vi "Calculate Assign Pt Demo.vi"(8 "Deform Array":dbl[](array[numeric])=[1.0, 1.0, 1.0, 0.0, 0.0, 0.0, 0.0, 0.0, 0.0], 9 "Eye Model Cluster":T2={"X Grid"=[], "Y Grid"=[], "Za_true Surf"=[], "Iris Center"=[], "Zp_true Surf"=[], "Pinv"=[[1.0, 0.0], [0.0, 1.0]], "za_true"=5.0, "za_work"=1.0, "zp_work"=-1.0, "zp_true"=-5.0}, 10 "Assign Pt":dbl[](array[numeric])=[0.0, 5.0, 0.0], 11 "Current Pt":dbl[](array[numeric])=[0.0, 0.0, 0.0]) -> (0 "Assign Pt OOB":bool, 3 "Assign Pt*":dbl[](array[numeric]))   [LabVIEW 2016]
uses:
  <vilib>/Analysis/Matrix/Datatypes/RealMatrix.ctl
  <vilib>/Analysis/_algsub.llb/Vector Norm Type.ctl
  <vilib>/Analysis/baseanly.llb/A x Vector.vi
  <vilib>/Analysis/_algsub.llb/Real Vector Norm.vi
  Subsystems/Global Variables.vi
  <vilib>/Analysis/7linalg.llb/Create Special Real Matrix.vi
  <vilib>/Analysis/baseanly.llb/Real Inverse Matrix.vi
  <vilib>/Analysis/NI_AALBase.lvlib
  <vilib>/Analysis/NI_AALPro.lvlib
  <vilib>/Analysis/NI_AALBLAS.lvlib
  <vilib>/Analysis/Matrix/NI_Matrix.lvlib
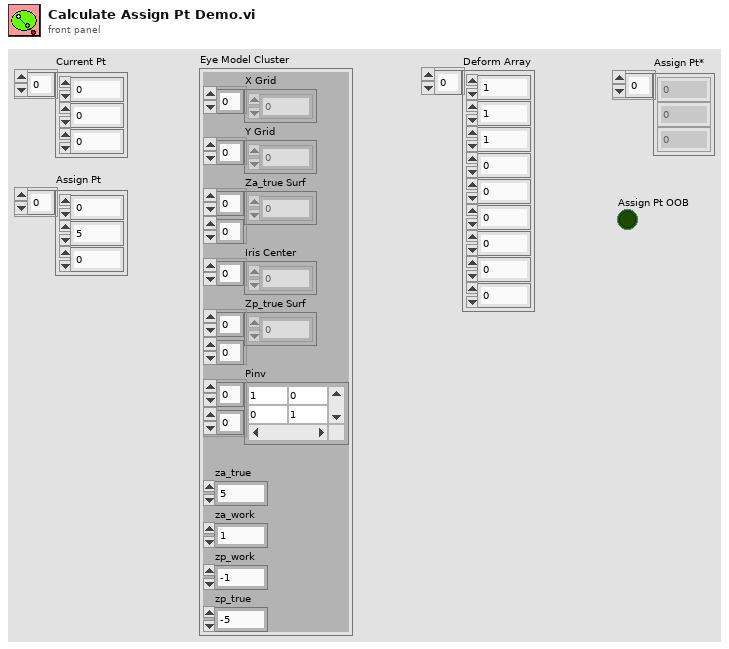
[diagram p1: front panel]
types:
  T1 = typedef "NI_Matrix.lvlib/RealMatrix.ctl" = dbl[][]
  T2 = cluster{"X Grid":dbl[], "Y Grid":dbl[], "Za_true Surf":dbl[][], "Iris Center":dbl[], "Zp_true Surf":dbl[][], "Pinv":T1, "za_true":dbl, "za_work":dbl, "zp_work":dbl, "zp_true":dbl}
  T3 = typedef "NI_AALPro.lvlib/Vector Norm Type.ctl" = u16
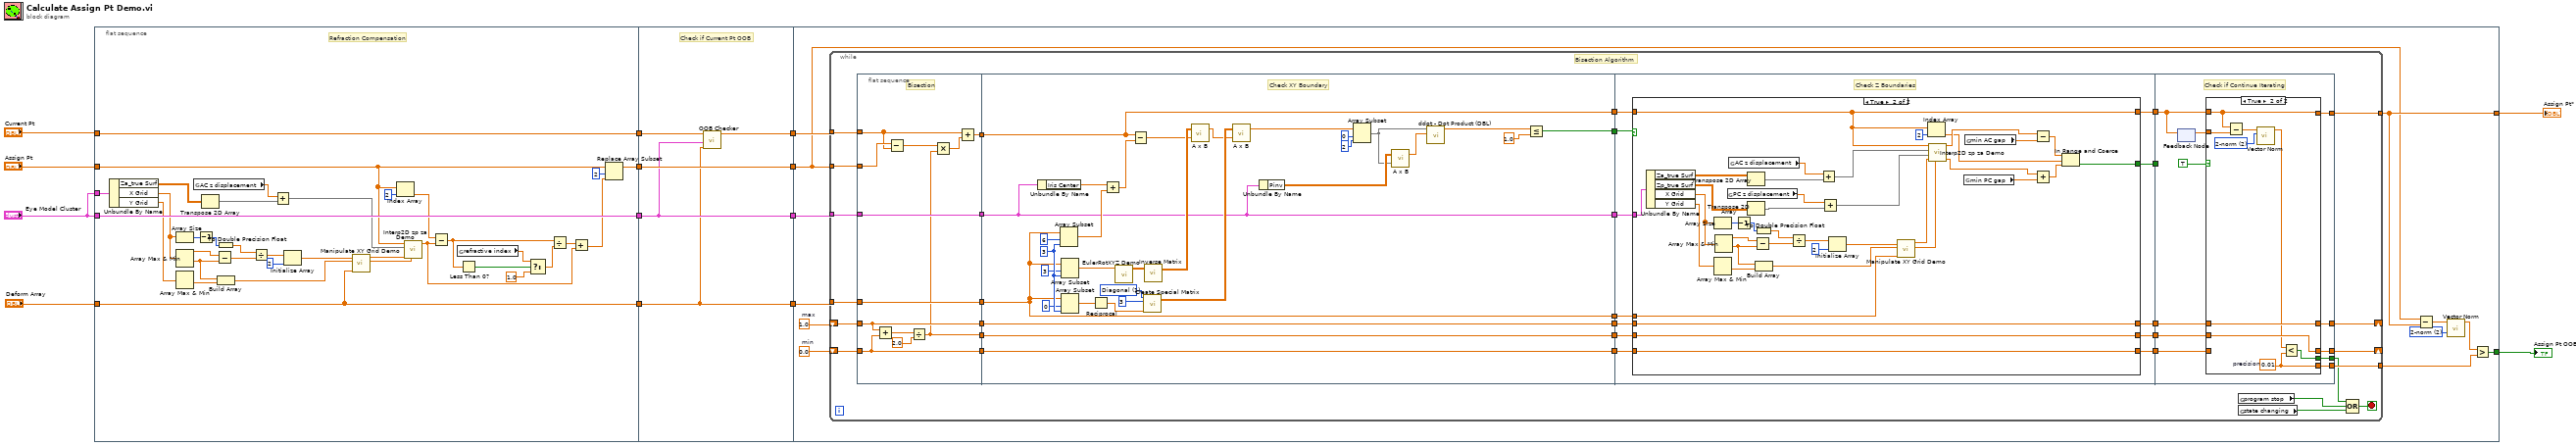
[diagram p0: block diagram]
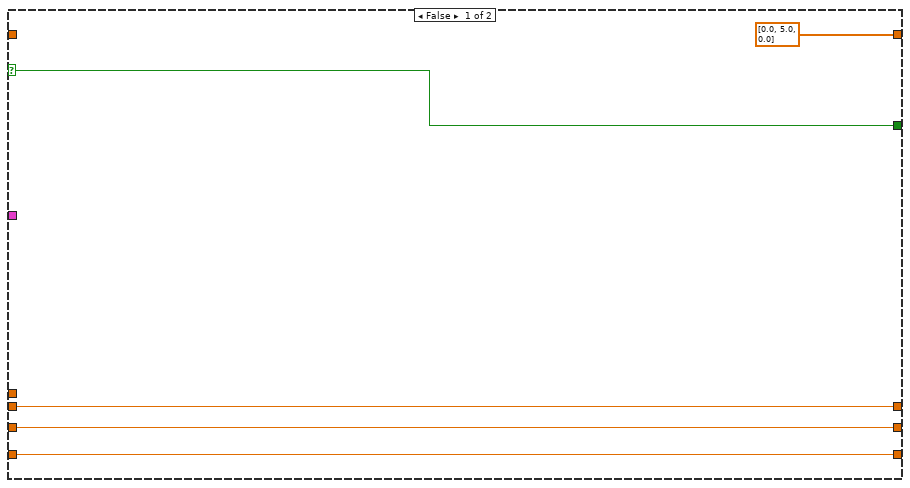
[diagram p2: hidden frame]
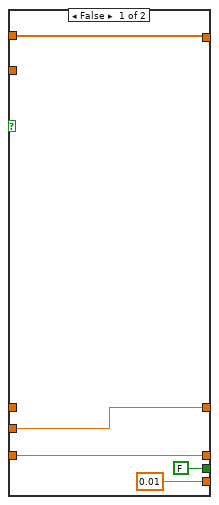
[diagram p3: hidden frame]
diagram:
  n1 = flat-sequence {
    tunnel: "Current Pt" -> [w28]
    tunnel: "Deform Array" -> [w30]
    tunnel: "Eye Model Cluster" -> [w50]
    tunnel: "Assign Pt" -> [w22]
    tunnel: [w23] -> w9
    tunnel: [w50] -> w7
    tunnel: [w30] -> w5
    tunnel: [w28] -> w3
    tunnel: "Eye Model Cluster" -> [w31]
    tunnel: w9 -> [w55]
    tunnel: [w55] -> w8
    tunnel: w7 -> [w52]
    tunnel: [w52] -> w6
    tunnel: w5 -> [w51]
    tunnel: [w51] -> w4
    tunnel: w3 -> [w54]
    tunnel: [w53] -> w2
    tunnel: w8 -> [w57]
    tunnel: w6 -> [w66]
    tunnel: w4 -> [w65]
    tunnel: w2 -> [w64]
    tunnel: [w60] -> w10
    tunnel: [w61] -> w1
    frame #0 {
      # "Refraction Compensation"
      n2 = Unbundle By Name(w31) -> ("Za_true Surf"=w34:dbl[][], "X Grid"=w46:dbl[], "Y Grid"=w47:dbl[])
      n3 = Array Size(array=w46) -> (size(s)=w39:i32)
      n4 = Array Max & Min(array=w46) -> (max value=w41:dbl, min value=w40:dbl)  [unwired: 2 out]
      n5 = Array Max & Min(array=w47) -> (min value=w42:dbl)  [unwired: 3 out]
      n6 = global read "Global Variables.vi" "AC z displacement"() -> (w33:dbl)
      n7 = Decrement(x=w39) -> (x-1=w44:i32)
      n8 = Transpose 2D Array(2D array=w34) -> (transposed array=w32:dbl[][])
      n9 = Subtract(x=w41, y=w40) -> (x-y=w45:dbl)
      n10 = To Double Precision Float(number=w44) -> (double precision float=w43:dbl)
      n11 = Build Array(w40, w42) -> (w35:dbl[])
      n12 = Divide(x=w43, y=w45) -> (x/y=w37:dbl)
      n13 = Add(x=w33, y=w32) -> (x+y=w29:dbl[][])
      n14 = Initialize Array(w37, 2 ("dimension size")) -> (w36:dbl[])
      n15 = call "Manipulate XY Grid Demo.vi"("Deform Array"=w30, "XY Grid min In"=w35, "XY Quant. Fact. In"=w36) -> ("XY Grid min Out"=w49:dbl[], "XY Quant. Fact. Out"=w48:dbl[])  [unwired: 7 in]
      n16 = Index Array(array=w22, index=2) -> (element=w26:dbl)
      n17 = call "Interp2D zp za Demo.vi"("XY Grid min"=w49, "XY Quantization Factor"=w48, "Za array"=w29, "Tip Position"=w22) -> ("za"=w25:dbl)  [unwired: 6 in, 1 out]
      n18 = Subtract(x=w26, y=w25) -> (x-y=w16:dbl)
      n19 = global read "Global Variables.vi" "refractive index"() -> (w18:dbl)
      n20 = Less Than 0?(x=w16) -> (x < 0?=w19:bool)
      n21 = Select(t=w18, s=w19, f=1.0) -> (s? t:f=w15:dbl)
      n22 = Divide(x=w16, y=w15) -> (x/y=w24:dbl)
      n23 = Add(x=w24, y=w25) -> (x+y=w20:dbl)
      n24 = Replace Array Subset(array=w22, new element=w20, index=2) -> (w23:dbl[])
    }
    frame #1 {
      # "Check if Current Pt OOB"
      n25 = call "OOB Checker.vi"("Deform Array"=w51, "Eye Model Cluster"=w52, "Check Pt"=w54) -> ("Check Pt*"=w53:dbl[])  [unwired: 7 in, 1 out]
    }
    frame #2 {
      w58 = T3 2 items=["1-norm"=1, "2-norm"=2, "Inf-norm"=3, "-Inf-norm"=4, "User Defined"=5] ("norm type")
      w67 = 0.0  # min
      w63 = 1.0  # max
      n26 = while {
        tunnel: w64 -> [w97]
        shift-right: [w80] -> _
        shift-left: w63 -> [w99]
        shift-right: [w78] -> _
        shift-left: w67 -> [w98]
        tunnel: w57 -> [w96]
        tunnel: w66 -> [w91]
        tunnel: w65 -> [w90]
        tunnel: [w73] -> w60
        tunnel: [w72] -> w62
        stop <- w71 stop-if-true
        # "Bisection Algorithm"
        n27 = flat-sequence {
          tunnel: [w107] -> w95
          tunnel: [w104] -> w94
          tunnel: [w103] -> w93
          tunnel: [w102] -> w92
          tunnel: [w101] -> w89
          tunnel: w99 -> [w104]
          tunnel: w98 -> [w103]
          tunnel: w97 -> [w108]
          tunnel: w96 -> [w109]
          tunnel: w91 -> [w102]
          tunnel: w90 -> [w101]
          tunnel: [w100] -> w77
          tunnel: w95 -> [w115]
          tunnel: w94 -> [w122]
          tunnel: w93 -> [w121]
          tunnel: w92 -> [w114]
          tunnel: w89 -> [w113]
          tunnel: [w123] -> w88
          tunnel: [w122] -> w87
          tunnel: [w121] -> w86
          tunnel: [w115] -> w85
          tunnel: [w114] -> w84
          tunnel: [w113] -> w83
          tunnel: w77 -> [w112]
          tunnel: [w112] -> w76
          tunnel: w88 -> [w155]
          tunnel: w87 -> [w154]
          tunnel: w86 -> [w153]
          tunnel: w85 -> [w151]
          tunnel: w84 -> [w152]
          tunnel: w83 -> [w150]
          tunnel: [w149] -> w82
          tunnel: [w148] -> w81
          tunnel: [w147] -> w79
          tunnel: w76 -> [w146]
          tunnel: [w145] -> w75
          tunnel: [w144] -> w74
          tunnel: w82 -> [_]
          tunnel: w81 -> [w209]
          tunnel: [w208] -> w80
          tunnel: w79 -> [w207]
          tunnel: [w206] -> w78
          tunnel: w75 -> [w205]
          tunnel: [w204] -> w70
          tunnel: w74 -> [w201]
          tunnel: [w203] -> w73
          tunnel: [w202] -> w72
          frame #0 {
            # "Bisection"
            n28 = Add(x=w104, y=w103) -> (x+y=w105:dbl)
            n29 = Subtract(x=w109, y=w108) -> (x-y=w111:dbl[])
            n30 = Divide(x=w105, y=2.0) -> (x/y=w100:dbl)
            n31 = Multiply(x=w111, y=w100) -> (x*y=w110:dbl[])
            n32 = Add(x=w108, y=w110) -> (x+y=w107:dbl[])
          }
          frame #1 {
            w132 = 1 items=["Identity", "Diagonal", "Toeplitz", "Vandermonde", "Companion", "Hankel", "Hadamard", "Wilkinson", "Hilbert", "Inverse Hilbert", "Rosser", "Pascal"] ("matrix type")
            w142 = 3 ("length")
            # "Check XY Boundary"
            n33 = Unbundle By Name(w114) -> ("Iris Center"=w129:dbl[])
            n34 = Array Subset(array=w113, index=6 ("length"), length=w142) -> (w128:dbl[])
            n35 = Array Subset(array=w113, index=3, length=w142) -> (w139:dbl[])
            n36 = Array Subset(array=w113, index=0, length=w142) -> (w135:dbl[])
            n37 = Reciprocal(x=w135) -> (1/x=w134:dbl[])
            n38 = Add(x=w129, y=w128) -> (x+y=w127:dbl[])
            n39 = call "EulerRotXYZ Demo.vi"("Euler Angle (XYZ)"=w139) -> ("Rotation Mtx"=w138:T1)  [unwired: 10 in]
            n40 = Subtract(x=w115, y=w127) -> (x-y=w136:dbl[])
            n41 = call-poly <vilib>:"Create Special Matrix.vi"("matrix type"=w132, "matrix size"=3, "Input Vector1"=w134) -> ("Special Matrix"=w131:T1)  [unwired: 2 in, 1 out]
            n42 = call-poly <vilib>:"Inverse Matrix.vi"("Input Matrix"=w138) -> ("Inverse Matrix"=w137:T1)  [unwired: 1 in, 1 out]
            n43 = call-poly <vilib>:"A x B.vi"("Vector"=w136, "A"=w137) -> ("A x Vector"=w130:dbl[])  [unwired: 1 out]
            n44 = call-poly <vilib>:"A x B.vi"("Vector"=w130, "A"=w131) -> ("A x Vector"=w120:dbl[])  [unwired: 1 out]
            n45 = Unbundle By Name(w114) -> ("Pinv"=w117:T1)
            n46 = Array Subset(array=w120, index=0, length=2) -> (w116:dbl[])
            n47 = call-poly <vilib>:"A x B.vi"("Vector"=w116, "A"=w117) -> ("A x Vector"=w126:dbl[])  [unwired: 1 out]
            n48 = call <vilib>:"ddot - Dot Product (DBL).vi"("y"=w126, "x"=w116) -> ("ddot"=w125:dbl)  [unwired: 8 in, 1 out]
            n49 = Less Or Equal?(x=w125, y=1.0) -> (x <= y?=w123:bool)
          }
          frame #2 {
            # "Check Z Boundaries"
            n50 = case shown="True" w155 {
              selector: w155 -> [w160 _]
              tunnel: w154 -> [w159 w164]
              tunnel: w153 -> [w157 w163]
              tunnel: w152 -> [_ w191]
              tunnel: w151 -> [_ w161]
              tunnel: w150 -> [_ w184]
              tunnel: [w160 w165] -> w149
              tunnel: [w159 w164] -> w148
              tunnel: [w157 w163] -> w147
              tunnel: [w158 w162] -> w145
              tunnel: w146 -> [w158 w162]
              tunnel: [dbl[] [0.0, 5.0, 0.0] w161] -> w144
              frame False {
              }
              frame True {
                n51 = Unbundle By Name(w191) -> ("Za_true Surf"=w177:dbl[][], "Zp_true Surf"=w175:dbl[][], "X Grid"=w190:dbl[], "Y Grid"=w189:dbl[])
                n52 = Array Size(array=w190) -> (size(s)=w192:i32)
                n53 = Array Max & Min(array=w189) -> (min value=w195:dbl)  [unwired: 3 out]
                n54 = Array Max & Min(array=w190) -> (max value=w194:dbl, min value=w193:dbl)  [unwired: 2 out]
                n55 = global read "Global Variables.vi" "PC z displacement"() -> (w182:dbl)
                n56 = global read "Global Variables.vi" "AC z displacement"() -> (w183:dbl)
                n57 = Decrement(x=w192) -> (x-1=w197:i32)
                n58 = Transpose 2D Array(2D array=w177) -> (transposed array=w176:dbl[][])
                n59 = Transpose 2D Array(2D array=w175) -> (transposed array=w174:dbl[][])
                n60 = Subtract(x=w194, y=w193) -> (x-y=w198:dbl)
                n61 = To Double Precision Float(number=w197) -> (double precision float=w196:dbl)
                n62 = Build Array(w193, w195) -> (w185:dbl[])
                n63 = Divide(x=w196, y=w198) -> (x/y=w187:dbl)
                n64 = Add(x=w183, y=w176) -> (x+y=w181:dbl[][])
                n65 = Add(x=w182, y=w174) -> (x+y=w180:dbl[][])
                n66 = Initialize Array(w187, 2 ("dimension size")) -> (w186:dbl[])
                n67 = call "Manipulate XY Grid Demo.vi"("Deform Array"=w184, "XY Grid min In"=w185, "XY Quant. Fact. In"=w186) -> ("XY Grid min Out"=w178:dbl[], "XY Quant. Fact. Out"=w179:dbl[])  [unwired: 7 in]
                n68 = Index Array(array=w161, index=2) -> (element=w166:dbl)
                n69 = call "Interp2D zp za Demo.vi"("XY Grid min"=w178, "XY Quantization Factor"=w179, "Zp array"=w180, "Za array"=w181, "Tip Position"=w161) -> ("zp"=w169:dbl, "za"=w170:dbl)  [unwired: 5 in]
                n70 = global read "Global Variables.vi" "min PC gap"() -> (w171:dbl)
                n71 = global read "Global Variables.vi" "min AC gap"() -> (w172:dbl)
                n72 = Subtract(x=w170, y=w172) -> (x-y=w168:dbl)
                n73 = Add(x=w169, y=w171) -> (x+y=w167:dbl)
                n74 = In Range and Coerce(upper limit=w168, x=w166, lower limit=w167) -> (In Range?=w165:bool)  [unwired: 1 out]
              }
            }
          }
          frame #3 {
            # "Check if Continue Iterating"
            n75 = feedback #1() -> (w200:dbl[])  [unwired: 1 in]
            n76 = feedback-in #1(w201) -> ()
            n77 = case shown="True" TRUE {
              tunnel: w209 -> [_ w223]
              tunnel: [w214 w223] -> w208
              tunnel: w207 -> [w213 _]
              tunnel: [w213 w222] -> w206
              tunnel: w205 -> [w214 w222]
              tunnel: [FALSE w221] -> w204
              tunnel: w201 -> [w210 w219]
              tunnel: [w210 w219] -> w203
              tunnel: [0.01 ("precision") w220] -> w202
              tunnel: w200 -> [_ w218]
              frame False {
              }
              frame True {
                w216 = T3 2 items=["1-norm"=1, "2-norm"=2, "Inf-norm"=3, "-Inf-norm"=4, "User Defined"=5] ("norm type")
                w220 = 0.01  # precision
                n78 = Subtract(x=w219, y=w218) -> (x-y=w217:dbl[])
                n79 = call-poly <vilib>:"Vector Norm.vi"("norm type"=w216, "Input Vector"=w217) -> ("norm"=w215:dbl)  [unwired: 8 in, 1 out]
                n80 = Less?(x=w215, y=w220) -> (x < y?=w221:bool)
              }
            }
          }
        }
        n81 = global read "Global Variables.vi" "program stop"() -> (w69:bool)
        n82 = global read "Global Variables.vi" "state changing"() -> (w68:bool)
        n83 = Compound Arithmetic op=OR(w70, w69, w68) -> (w71:bool)
      }
      n84 = Subtract(x=w57, y=w60) -> (x-y=w59:dbl[])
      n85 = call-poly <vilib>:"Vector Norm.vi"("norm type"=w58, "Input Vector"=w59) -> ("norm"=w56:dbl)  [unwired: 8 in, 1 out]
      n86 = Greater?(x=w56, y=w62) -> (0:w61:bool)
    }
  }
  "Assign Pt*" <- w10
  "Assign Pt OOB" <- w1
